vi "Save Report to File.vi"(0 "report in":refnum<class "NI_report.lvclass">, 5 "report file path":path, 7 "prompt to replace? (F)":bool, 9 "password (\"\")":string, 11 "error in (no error)":errorcluster) -> (4 "report out":refnum<class "NI_report.lvclass">, 15 "error out":errorcluster)   [LabVIEW 2015, in "NI_report.lvclass"]
doc: "Saves an HTML report to the file specified in <B>report file path</B>. You cannot use this VI with standard reports.\n\nThis VI also saves Microsoft Word and Excel reports."
uses:
  <vilib>/Utility/NIReport.llb/NI_report.lvclass
  <vilib>/Utility/NIReport.llb/NI_ReportGenerationCore.lvlib
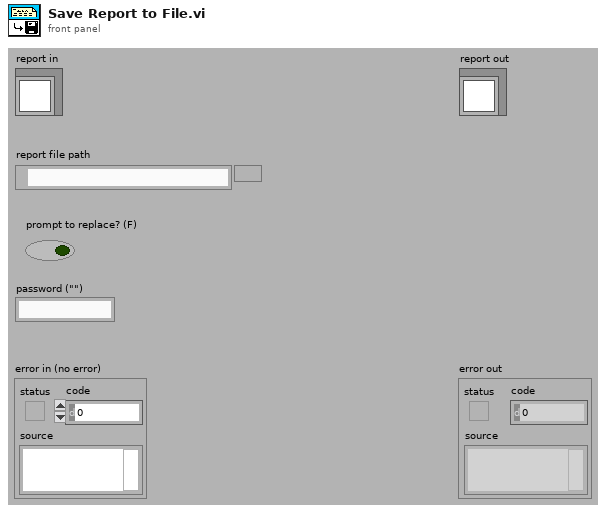
[diagram p1: front panel]
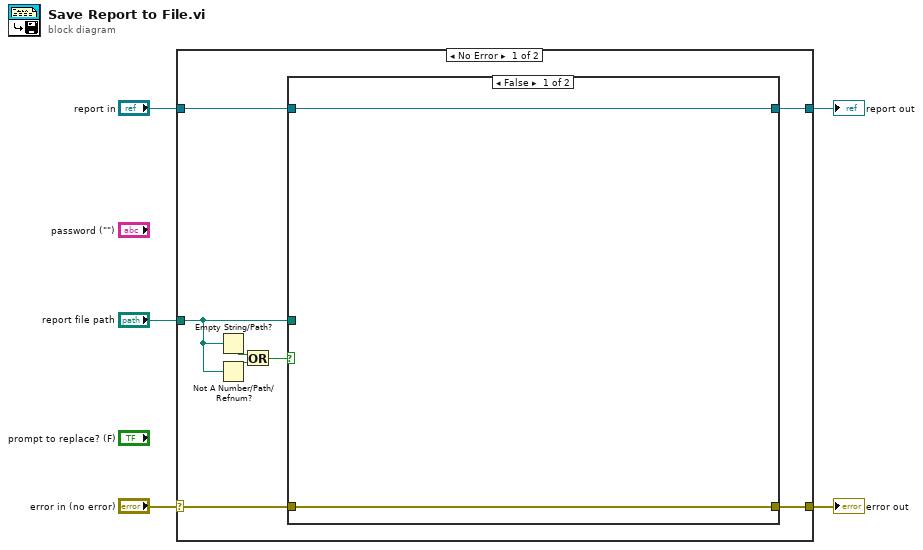
[diagram p0: block diagram]
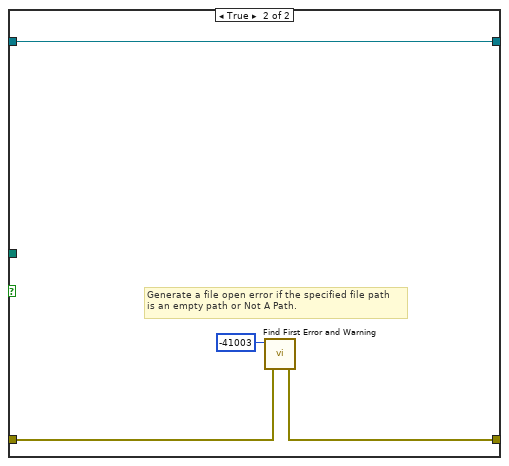
[diagram p2: hidden frame]
diagram:
  n1 = case shown="No Error" "error in (no error)" {
    selector: "error in (no error)" -> [w7 w21]
    tunnel: [w8 w20] -> w3
    tunnel: "report in" -> [w9 w20]
    tunnel: "report file path" -> [w10 _]
    tunnel: [w6 w21] -> w1
    frame No Error {
      n2 = Empty String/Path?(string/path=w10) -> (empty?=w12:bool)
      n3 = Not A Number/Path/Refnum?(number/path/refnum=w10) -> (NaN/Path/Refnum?=w11:bool)
      n4 = Or(x=w12, y=w11) -> (x .or. y?=w13:bool)
      n5 = case shown="False" w13 {
        tunnel: [w15 w19] -> w8
        tunnel: w9 -> [w15 w19]
        tunnel: w10 -> [_ _]
        tunnel: w7 -> [w14 w17]
        tunnel: [w14 w16] -> w6
        frame False {
        }
        frame True {
          # "Generate a file open error if the specified file path\nis an empty path or Not A Path."
          n6 = call <vilib>:"Find First Error and Warning.vi"("error in (no error)"=w17, "error code"=-41003) -> ("error out"=w16:errorcluster)  [unwired: 1 in, 4 out]
        }
      }
    }
    frame Error {
    }
  }
  "error out" <- w1
  "report out" <- w3
